vi "part2.vi"() -> ()   [LabVIEW 2009]
panel:
  out "Array":bool[](array[boolean])
  in  "stop":bool
  # "TTL input from 4 dipswitches"
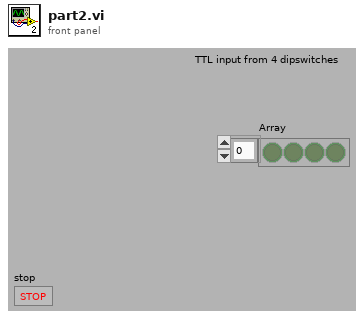
[diagram p1: front panel]
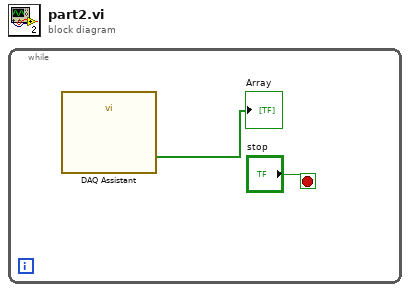
[diagram p0: block diagram]
diagram:
  n1 = while {
    stop <- "stop" stop-if-true
    n2 = call "DAQ Assistant"() -> ("data"=→"Array":bool[])  [unwired: 17 in, 2 out]
  }
